vi "Inverse Hilbert Matrix (DBL).vi"(11 "matrix size":i32) -> (0 "error":i32, 3 "Inverse Hilbert Matrix":T1)   [LabVIEW 2020, in "NI_AALPro.lvlib"]
uses:
  NI_AALPro.lvlib
  RealMatrix.ctl
  NI_Gmath.lvlib
  NI_Matrix.lvlib
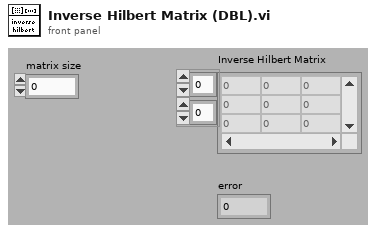
[diagram p1: front panel]
types:
  T1 = typedef "NI_Matrix.lvlib/RealMatrix.ctl" = dbl[][]
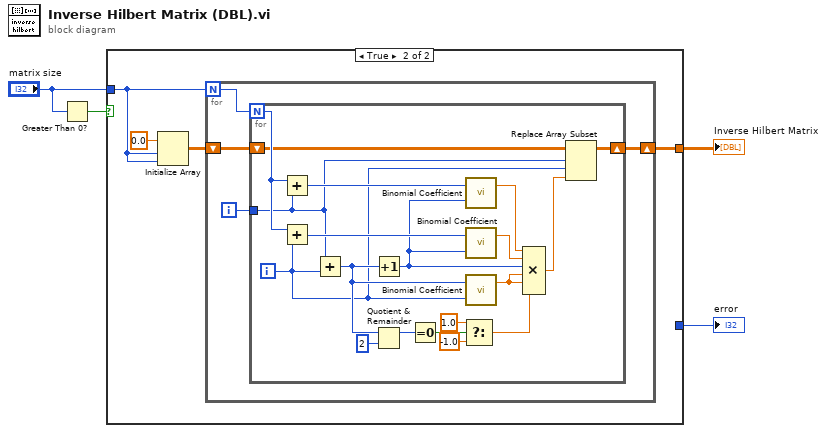
[diagram p0: block diagram]
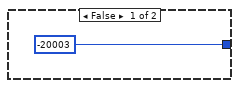
[diagram p2: hidden frame]
diagram:
  n1 = Greater Than 0?(x="matrix size") -> (x > 0?=w3:bool)
  n2 = case shown="True" w3 {
    tunnel: [_ w9] -> w1
    tunnel: [-20003 _] -> w4
    tunnel: "matrix size" -> [_ w6]
    frame False {
    }
    frame True {
      n3 = Initialize Array(0.0 ("element"), w6, w6) -> (w8:dbl[][])
      n4 = for {
        N: w6 -> [w12]
        shift-right: [w10] -> w9
        shift-left: w8 -> [w11]
        i -> [w13]
        n5 = for {
          N: w12 -> [w24]
          tunnel: w13 -> [w15]
          shift-right: [w17] -> w10
          shift-left: w11 -> [w18]
          i -> [w14]
          n6 = Add(x=w24, y=w15) -> (x+y=w23:i32)
          n7 = Add(x=w24, y=w14) -> (x+y=w22:i32)
          n8 = Add(x=w15, y=w14) -> (x+y=w25:i32)
          n9 = Increment(x=w25) -> (x+1=w21:i32)
          n10 = Quotient & Remainder(x=w25, y=2) -> (x-y*floor(x/y)=w29:i32)  [unwired: 1 out]
          n11 = Equal To 0?(x=w29) -> (x = 0?=w28:bool)
          n12 = Select(t=1.0, s=w28, f=-1.0 ("t")) -> (s? t:f=w19:dbl)
          n13 = call "Binomial Coefficient.vi"("k"=w21, "n"=w23) -> ("binomial coefficient (n,k)"=w31:dbl)  [unwired: 1 out]
          n14 = call "Binomial Coefficient.vi"("k"=w21, "n"=w22) -> ("binomial coefficient (n,k)"=w32:dbl)  [unwired: 1 out]
          n15 = call "Binomial Coefficient.vi"("k"=w14, "n"=w25) -> ("binomial coefficient (n,k)"=w20:dbl)  [unwired: 1 out]
          n16 = Compound Arithmetic op=MULTIPLY(w31, w32, w21, w20, w20, w19) -> (w16:dbl)
          n17 = Replace Array Subset(array=w18, new element=w16, index (row)=w15, index (col)=w14) -> (w17:dbl[][])
        }
      }
    }
  }
  "error" <- w4
  "Inverse Hilbert Matrix" <- w1
